vi "ACQ Create counter tasks.vi"(4 "frequency (100000Hz)":dbl=100000.0 format="%#_13g", 6 "device in":tag="Dev1", 7 "Config Counter channels":T3, 8 "error in (no error)":errorcluster, 11 "All Read tasks in":T2) -> (0 "error out":errorcluster, 2 "Tasks ref out":T1, 3 "All Read tasks out":T2)   [LabVIEW 2013]
doc: "Konfiguruje kanały licznikow:\n2 liczniki wejściowe Enkoder X, Enkoder Y\n1 generator freqout\nwybiera wyjście generatora OUT"
uses:
  Kontrolki/KartaDAQ/ACQ counter channel config.ctl
  Kontrolki/KartaDAQ/ACQ all read tasks.ctl
  Kontrolki/KartaDAQ/ACQ Counter refnum.ctl
  <vilib>/DAQmx/create/channels.llb/DAQmx Create Channel (CI-Position-Linear Encoder).vi
  <vilib>/DAQmx/create/channels.llb/DAQmx Create Channel (CO-Pulse Generation-Frequency).vi
  <resource>/objmgr/daqmx.rc
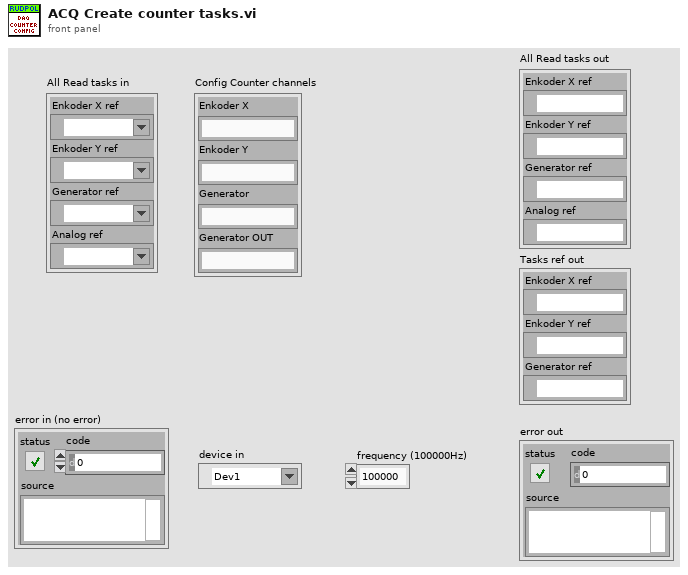
[diagram p1: front panel]
types:
  T1 = typedef "ACQ Counter refnum.ctl" = cluster{"Enkoder X ref":refnum<k21>, "Enkoder Y ref":refnum<k21>, "Generator ref":refnum<k21>}
  T2 = typedef "ACQ all read tasks.ctl" = cluster{"Enkoder X ref":refnum<k21>, "Enkoder Y ref":refnum<k21>, "Generator ref":refnum<k21>, "Analog ref":refnum<k21>}
  T3 = typedef "ACQ counter channel config.ctl" = cluster{"Enkoder X":string, "Enkoder Y":string, "Generator":string, "Generator OUT":string}
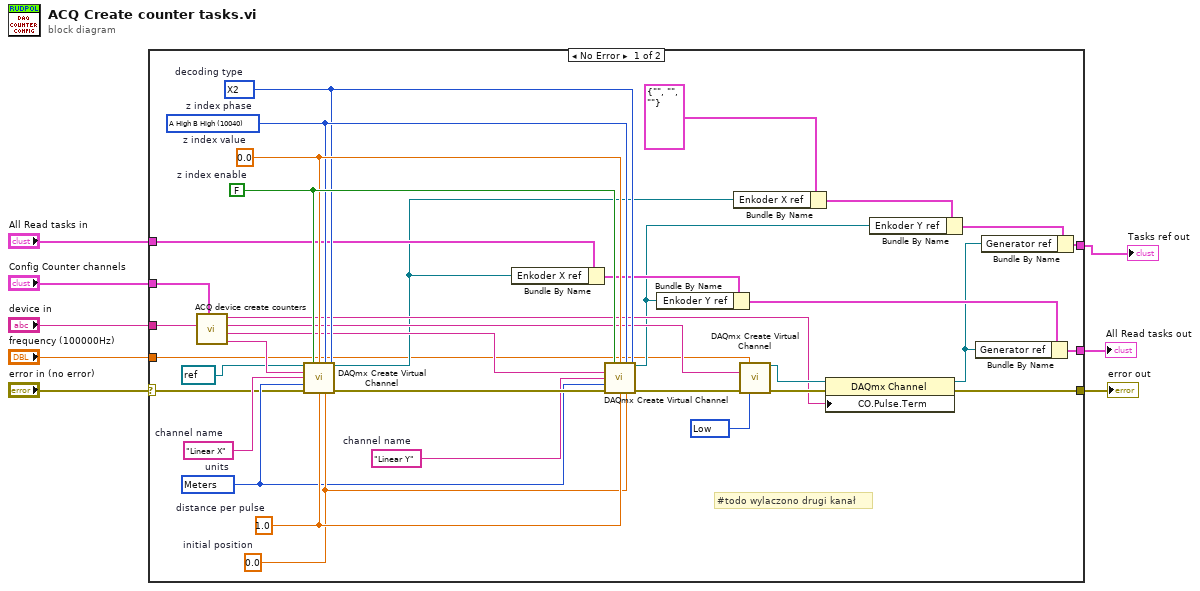
[diagram p0: block diagram]
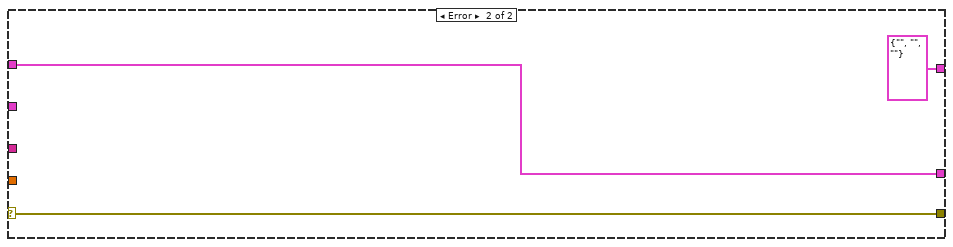
[diagram p2: hidden frame]
diagram:
  n1 = case shown="No Error" "error in (no error)" {
    selector: "error in (no error)" -> [w19 w46]
    tunnel: [w33 w46] -> w8
    tunnel: [w26 w45] -> w3
    tunnel: "device in" -> [w25 _]
    tunnel: "Config Counter channels" -> [w24 _]
    tunnel: "All Read tasks in" -> [w18 w45]
    tunnel: [w15 T1 {"Enkoder X ref"="", "Enkoder Y ref"="", "Generator ref"=""} ("Tasks ref out")] -> w2
    tunnel: "frequency (100000Hz)" -> [w10 _]
    frame No Error {
      w37 = 1.0  # distance per pulse
      w34 = "Linear Y"  # channel name
      w35 = 10219 items=["Meters"=10219, "Inches"=10379, "Ticks"=10304, "From Custom Scale"=10065]  # units
      w39 = 10091 items=["X1"=10090, "X2"=10091, "X4"=10092, "Two Pulse Counting"=10313]  # decoding type
      w36 = 0.0  # initial position
      w40 = 10040 items=["A High B High"=10040, "A High B Low"=10041, "A Low B High"=10042, "A Low B Low"=10043]  # z index phase
      w41 = 0.0  # z index value
      w42 = FALSE  # z index enable
      w38 = "Linear X"  # channel name
      w32 = 10214 items=["High"=10192, "Low"=10214] ("idle state")
      # "#todo wylaczono drugi kanał"
      n2 = call "ACQ device create counters.vi"("Config Counter channels"=w24, "device in"=w25) -> ("DAQ en X"=w23:tag, "DAQ en Y"=w22:tag, "DAQ gen"=w21:tag, "DAQ gen out"=w20:tag)  [unwired: 6 in]
      n3 = call-poly <vilib>:"DAQmx Create Virtual Channel.vi"("task in"=refnum<k21> refnum, "z index enable"=w42, "z index value"=w41, "z index phase"=w40, "counter"=w23, "decoding type"=w39, "name to assign"=w38, "units"=w35, "error in"=w19, "distance per pulse"=w37, "initial position"=w36) -> ("task out"=w11:refnum<k21>, "error out"=w43:errorcluster)  [unwired: 3 in]
      n4 = Bundle By Name(cluster=w18, "Enkoder X ref"=w11) -> (w30:T2)
      n5 = call-poly <vilib>:"DAQmx Create Virtual Channel.vi"("z index enable"=w42, "z index value"=w41, "z index phase"=w40, "counter"=w22, "decoding type"=w39, "name to assign"=w34, "units"=w35, "error in"=w43, "distance per pulse"=w37, "initial position"=w36) -> ("task out"=w12:refnum<k21>, "error out"=w31:errorcluster)  [unwired: 4 in]
      n6 = Bundle By Name(cluster=w30, "Enkoder Y ref"=w12) -> (w29:T2)
      n7 = Bundle By Name(cluster=T1 {"Enkoder X ref"="", "Enkoder Y ref"="", "Generator ref"=""} ("Tasks ref out"), "Enkoder X ref"=w11) -> (w16:T1)
      n8 = call-poly <vilib>:"DAQmx Create Virtual Channel.vi"("frequency"=w10, "counter"=w21, "error in"=w31, "idle state"=w32) -> ("task out"=w28:refnum<k21>, "error out"=w27:errorcluster)  [unwired: 10 in]
      n9 = property class="DAQmx Channel"(reference=w28, error in=w27, "CO.Pulse.Term"=w20) -> (reference out=w13:refnum<k21>, error out=w33:errorcluster)
      n10 = Bundle By Name(cluster=w16, "Enkoder Y ref"=w12) -> (w14:T1)
      n11 = Bundle By Name(cluster=w29, "Generator ref"=w13) -> (w26:T2)
      n12 = Bundle By Name(cluster=w14, "Generator ref"=w13) -> (w15:T1)
    }
    frame Error {
    }
  }
  "error out" <- w8
  "All Read tasks out" <- w3
  "Tasks ref out" <- w2
